vi "Connect.vi"(8 "error in":errorcluster, 11 "ProXR_IO in":refnum<class "ProXR.lvclass">) -> (0 "error out":errorcluster, 3 "ProXR_IO out":refnum<class "ProXR.lvclass">)   [LabVIEW 2019, in "ProXR.lvlib" / "ProXR.lvclass"]
uses:
  Library/ProXR.lvclass
  C:/Users/Public/Documents/Development/builds/Instruments/Instruments.lvlibp/Library/Instruments.lvclass
  Library/ProXR.lvclass/ProXR.ctl
  builds/Instruments/Instruments.lvlibp/Accessors/Read Resource.vi
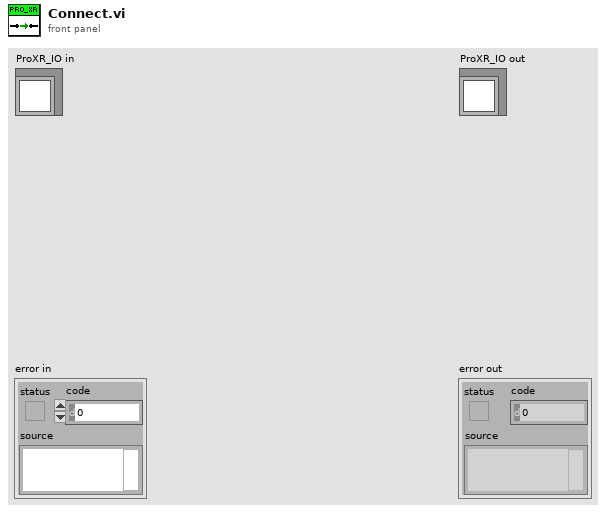
[diagram p1: front panel]
types:
  T1 = cluster{"Baud Rate":u32, "Parity":u16, "Data Bits":u16, "Stop Bits":u16, "Flow Control":u16}
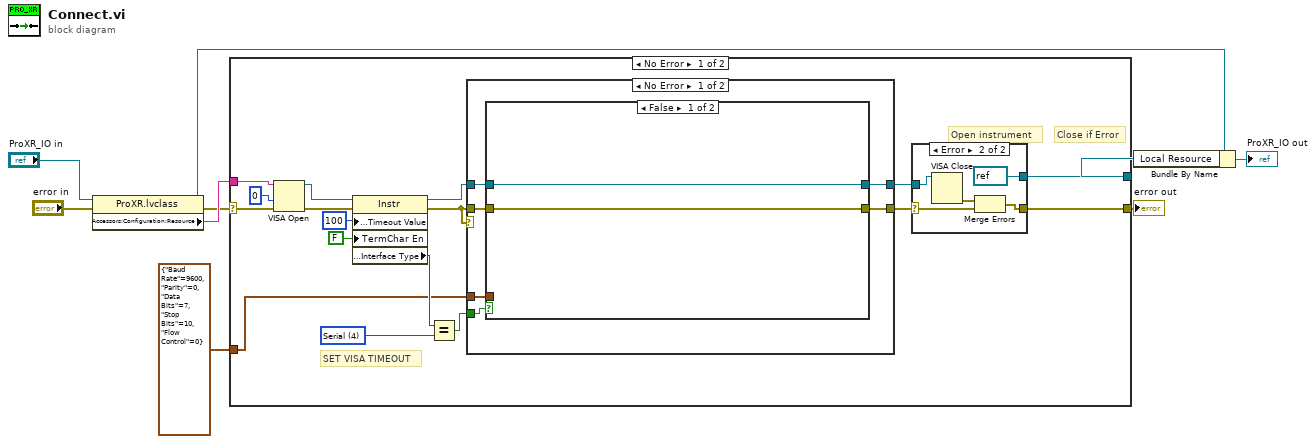
[diagram p0: block diagram]
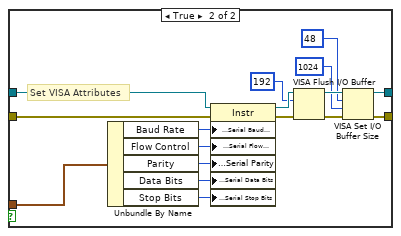
[diagram p2: hidden frame]
diagram:
  n1 = property class="ProXR.lvclass"(reference="ProXR_IO in", error in="error in") -> (reference out=w5:refnum<class "ProXR.lvclass">, error out=w6:errorcluster, "Accessors:Configuration:Resource"=w7:string)
  n2 = case shown="No Error" w6 {
    selector: w6 -> [w13 w62]
    tunnel: [w20 w61] -> w4
    tunnel: [w19 w62] -> w2
    tunnel: w7 -> [w12 w61]
    tunnel: T1 {"Baud Rate"=9600, "Parity"=0, "Data Bits"=7, "Stop Bits"=10, "Flow Control"=0} ("Serial Configuration") -> [w11 _]
    frame No Error {
      w22 = u16 4 items=["GPIB"=1, "VXI"=2, "GPIB-VXI"=3, "Serial"=4, "PXI"=5, "TCPIP"=6, "USB"=7] ("Interface Information:Interface Type")
      # "SET VISA TIMEOUT"
      # "Close if Error"
      # "Open instrument"
      n3 = VISA Open(access mode=u32 0, error in (no error)=w13, VISA resource name=w12) -> (VISA resource name=w16:refnum<visa-resource-name>, error out=w15:errorcluster)  [unwired: 2 in]
      n4 = property class="Instr"(reference=w16, error in=w15, "General Settings:Timeout Value"=u32 100, "TermChar En"=FALSE ("Message Based Settings:Termination Character Enable")) -> (reference out=w24:refnum<visa-resource-name>, error out=w14:errorcluster, "Interface Information:Interface Type"=w26:u16)
      n5 = Equal?(x=w26, y=w22) -> (x = y?=w23:bool)
      n6 = case shown="No Error" w14 {
        tunnel: w24 -> [w32 w53]
        tunnel: w14 -> [w31 w52]
        tunnel: w23 -> [w30 _]
        tunnel: [w29 w52] -> w18
        tunnel: [w28 w53] -> w17
        tunnel: w11 -> [w27 _]
        frame No Error {
          n7 = case shown="False" w30 {
            tunnel: [w33 w48] -> w28
            tunnel: [w34 w45] -> w29
            tunnel: w32 -> [w33 w50]
            tunnel: w31 -> [w34 w51]
            tunnel: w27 -> [_ w37]
            frame False {
            }
            frame True {
              # "Set VISA Attributes"
              n8 = Unbundle By Name(w37) -> ("Baud Rate"=w40:u32, "Flow Control"=w36:u16, "Parity"=w38:u16, "Data Bits"=w39:u16, "Stop Bits"=w35:u16)
              n9 = property class="Instr"(reference=w50, error in=w51, "Serial Settings:Serial Baud Rate"=w40, "Serial Settings:Serial Flow Control"=w36, "Serial Settings:Serial Parity"=w38, "Serial Settings:Serial Data Bits"=w39, "Serial Settings:Serial Stop Bits"=w35) -> (reference out=w44:refnum<visa-resource-name>, error out=w47:errorcluster)
              n10 = VISA Flush I/O Buffer(VISA resource name=w44, mask (16)=u16 192, error in (no error)=w47) -> (VISA resource name out=w49:refnum<visa-resource-name>, error out=w46:errorcluster)
              n11 = VISA Set I/O Buffer Size(VISA resource name=w49, mask (16)=u16 48, size (4096)=u32 1024 ("size (0)"), error in (no error)=w46) -> (VISA resource name out=w48:refnum<visa-resource-name>, error out=w45:errorcluster)
            }
          }
        }
        frame Error {
        }
      }
      n12 = case shown="Error" w18 {
        selector: w18 -> [w54 w56]
        tunnel: w17 -> [w55 w58]
        tunnel: [w55 refnum<visa-resource-name> refnum ("VISA resource name out")] -> w20
        tunnel: [w54 w57] -> w19
        frame No Error {
        }
        frame Error {
          n13 = VISA Close(VISA resource name=w58) -> (error out=w59:errorcluster)  [unwired: 1 in]
          n14 = Merge Errors(w59, w56) -> (w57:errorcluster)
        }
      }
    }
    frame Error {
    }
  }
  "error out" <- w2
  n15 = Bundle By Name(cluster=w5, "Local Resource"=w4) -> (→"ProXR_IO out":refnum<class "ProXR.lvclass">)
